vi "IMSCOM9.vi"() -> ()   [LabVIEW 2009]
uses:
  <vilib>/Instr/_visa.llb/VISA Configure Serial Port (Instr).vi
panel:
  out "Velocity":dbl
  in  "Go":bool
  in  "stop":bool
  in  "Move to":i32=-40000
  out "FP":string
  out "DETZ HIGH LIM":i32=-94296
  out "DETZ LOW LIM":i32=-34296
  out "COM PORT":refnum<visa-resource-name>="COM5"
  out "In Range?":bool
  out "Current Values":i32
  # "XES DETZ CONTROL"
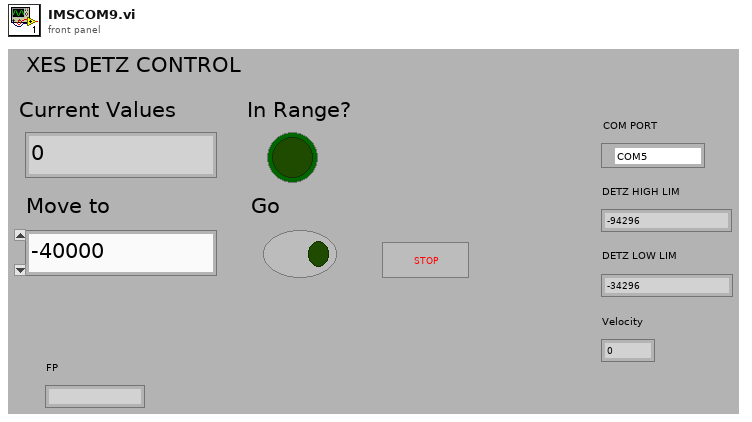
[diagram p1: front panel]
types:
  T1 = enum16{"Power-up Signature", "Accel Rate", "Accel Max", "Bit Rate", "Buffer Status", "Change Current", "Commence Jogging", "Change Jog Speed", "Continue", "Define Address", "Distance for FC,FM,FO,FY", "Decel Rate", "Distance or Position", "Define Limits", "Encoder Deadband", "Encoder Function", "Encoder Position", "Encoder Ratio", "Feed to Length with Speed Change", "Feed to Length", "Feed to Sensor with Mask Dist", "Feed to Length & Set Output", "Feed to Position", "Feed to Sensor", "Feed to Sensor w/safety", "Follow Handwheel", "Immediate Distance?", "Immediate Encoder?", "Immediate Low Output", "Immediate High Output", "Immediate Position?", "Input Status?", "Jog Accel/Decel", "Jog Disable", "Jog Enable", "Jog Speed", "Motor Disable", "Motor Enable", "Microstep Resolution", "Power up Current", "Power up Mode", "Pause", "Request Status", "Revision Level?", "Seek Home", "Stop Jogging", "Stop & Kill Buffer", "Set Output", "Set ABS Position", "Send String", "Stop", "Velocity for Speed Change", "Velocity Setting", "Wait for Input", "Wait Time"}
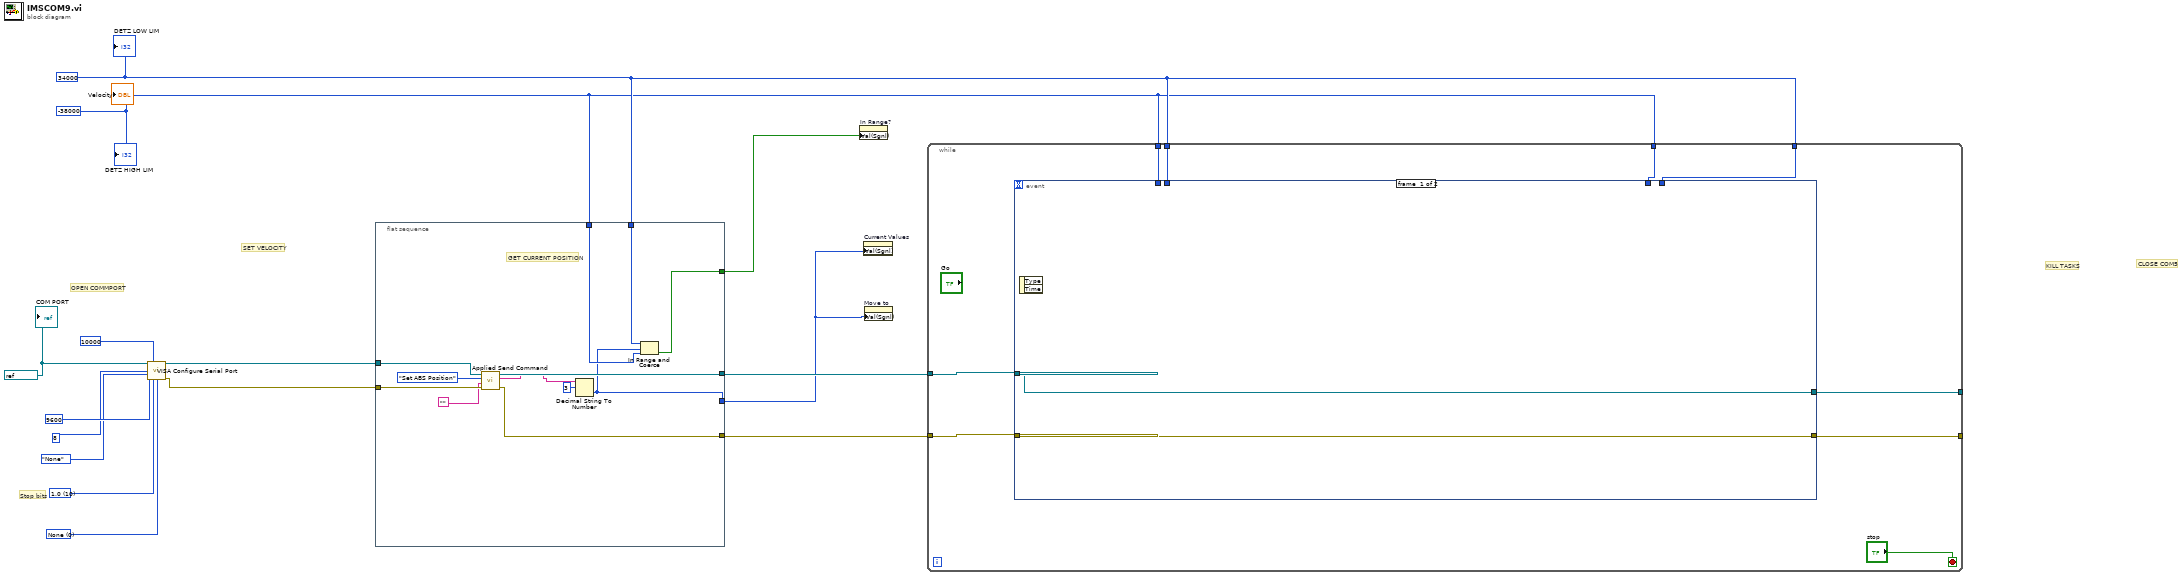
[diagram p0: block diagram]
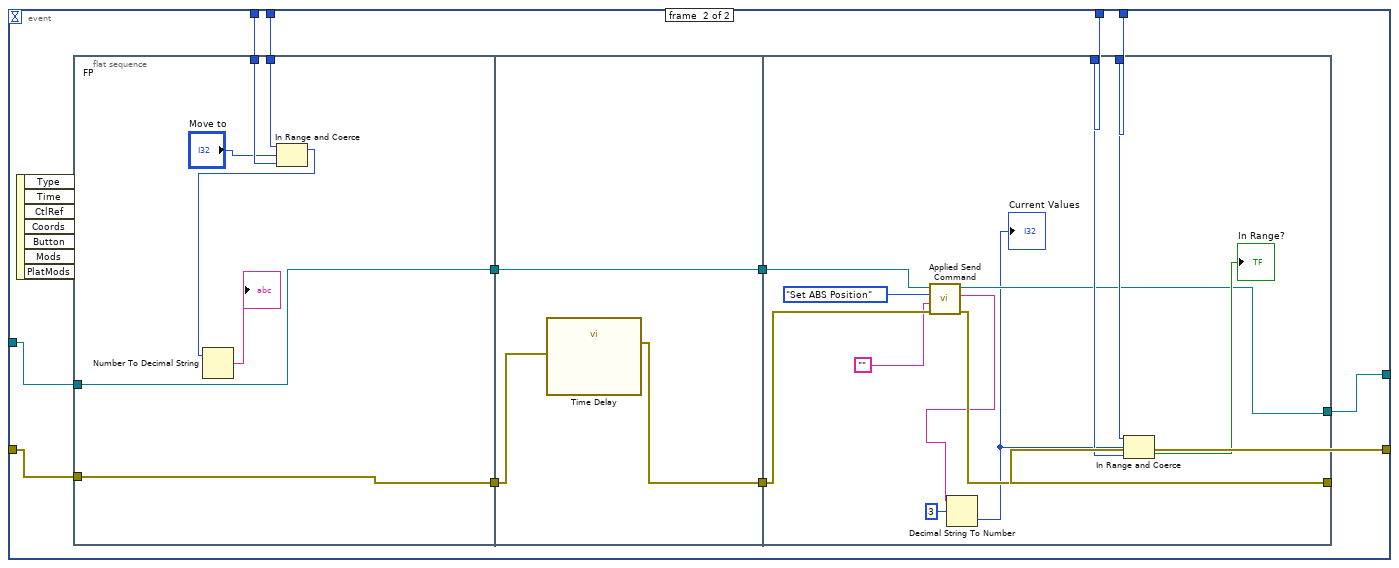
[diagram p2: hidden frame]
diagram:
  w1 = -38000 ("lower limit")
  w2 = 34000 ("upper limit")
  w7 = refnum<visa-resource-name> "COM5" ("COM PORT")
  w11 = u16 0 items=["None", "XON/XOFF", "RTS/CTS", "XON/XOFF & RTS/CTS", "DTR/DSR", "XON/XOFF & DTR/DSR"] ("flow control (0:none)")
  w12 = u16 10 items=["1.0"=10, "1.5"=15, "2.0"=20] ("stop bits (10: 1 bit)")
  # "CLOSE COM5"
  # "KILL TASKS"
  # "SET VELOCITY"
  # "Stop bits"
  # "OPEN COMMPORT"
  n1 = call-poly "VISA Configure Serial Port"("VISA resource name"=w7, "timeout (10sec)"=u32 10000, "baud rate (9600)"=u32 9600, "data bits (8)"=u16 8, "parity (0:none)"=enum16{"None", "Odd", "Even", "Mark", "Space"}."None", "stop bits (10: 1 bit)"=w12, "flow control (0:none)"=w11) -> ("VISA resource name out"=w8:refnum<visa-resource-name>, "error out"=w9:errorcluster)  [unwired: 7 in]
  n2 = flat-sequence {
    tunnel: w9 -> [w27]
    tunnel: w8 -> [w26]
    tunnel: w2 -> [w24]
    tunnel: w1 -> [w23]
    tunnel: [w25] -> w5
    tunnel: [w17] -> w4
    tunnel: [w22] -> w3
    tunnel: [w21] -> w6
    frame #0 {
      # "GET CURRENT POSITION"
      n3 = call "Applied Send Command.vi"("error in (no error)"=w27, "Extra"="", "Command"=T1."Set ABS Position", "VISA resource name"=w26) -> ("error out"=w25:errorcluster, "read buffer"=w19:string, "VISA resource name out"=w21:refnum<visa-resource-name>)  [unwired: 3 in]
      n4 = Decimal String To Number(string=w19, offset=3) -> (number=w17:i32)  [unwired: 1 in, 1 out]
      n5 = In Range and Coerce(upper limit=w24, x=w17, lower limit=w23) -> (In Range?=w22:bool)  [unwired: 1 out]
    }
  }
  n6 = property on="In Range?" class="Bool (strict)"("Val(Sgnl)"=w3) -> ()  [unwired: 2 in, 2 out]
  n7 = property on="Current Values" class="DigNum (strict)"("Val(Sgnl)"=w4) -> ()  [unwired: 2 in, 2 out]
  n8 = property on="Move to" class="DigNum (strict)"("Val(Sgnl)"=w4) -> ()  [unwired: 2 in, 2 out]
  n9 = while {
    tunnel: w6 -> [w32]
    tunnel: w5 -> [w31]
    tunnel: w1 -> [w35]
    tunnel: w2 -> [w34]
    tunnel: [w33] -> _
    tunnel: [w30] -> _
    tunnel: w2 -> [w29]
    tunnel: w1 -> [w28]
    stop <- "stop" stop-if-true
    n10 = event shown="[1] \"Go\": Mouse Up" {
      selector: _ -> [_ _]
      dyn-events: _ -> [_ _]
      timeout: _ -> [_ _]
      tunnel: w31 -> [w38 w47]
      tunnel: w35 -> [_ w50]
      tunnel: w34 -> [_ w49]
      tunnel: [w38 w48] -> w33
      tunnel: w32 -> [w37 w46]
      tunnel: [w37 w45] -> w30
      tunnel: w29 -> [_ w40]
      tunnel: w28 -> [_ w39]
      event #0 {
        n11 = event-data() -> ()  [unwired: 1 in, 2 out]
      }
      event #1 {
        n12 = event-data() -> ()  [unwired: 1 in, 7 out]
        n13 = flat-sequence {
          tunnel: [w56] -> w44
          tunnel: w47 -> [w56]
          tunnel: [w55] -> w42
          tunnel: w46 -> [w55]
          tunnel: w40 -> [w54]
          tunnel: w39 -> [w53]
          tunnel: w44 -> [w59]
          tunnel: [w58] -> w43
          tunnel: w42 -> [w60]
          tunnel: [w60] -> w41
          tunnel: w50 -> [w71]
          tunnel: w49 -> [w70]
          tunnel: [w69] -> w48
          tunnel: w43 -> [w68]
          tunnel: [w65] -> w45
          tunnel: w41 -> [w64]
          frame #0 {
            n14 = In Range and Coerce(upper limit=w54, x="Move to", lower limit=w53) -> (coerced(x)=w51:i32)  [unwired: 1 out]
            n15 = Number To Decimal String(number=w51) -> (decimal integer string=→"FP":string)  [unwired: 1 in]
          }
          frame #1 {
            n16 = call "Time Delay"("error in (no error)"=w59) -> ("error out"=w58:errorcluster)  [unwired: 10 in]
          }
          frame #2 {
            n17 = call "Applied Send Command.vi"("error in (no error)"=w68, "Extra"="", "Command"=T1."Set ABS Position", "VISA resource name"=w64) -> ("error out"=w69:errorcluster, "read buffer"=w67:string, "VISA resource name out"=w65:refnum<visa-resource-name>)  [unwired: 3 in]
            n18 = Decimal String To Number(string=w67, offset=3) -> (number=w63:i32)  [unwired: 1 in, 1 out]
            "Current Values" <- w63
            n19 = In Range and Coerce(upper limit=w70, x=w63, lower limit=w71) -> (In Range?=→"In Range?":bool)  [unwired: 1 out]
          }
        }
      }
    }
  }
  "COM PORT" <- w7
  "DETZ LOW LIM" <- w2
  "DETZ HIGH LIM" <- w1
